vi "READ PORT.vi"(6 "wait for reply (T)":bool=TRUE, 8 "error in (no error)":errorcluster, 10 "CANAL":u8, 11 "Module ID":i32=-1) -> (0 "error out":errorcluster, 1 "timed out?":bool, 2 "Reply Payload":T1)   [LabVIEW 2019, in "MAIN.lvlib"]
doc: "LEE EL PUERTO COMPLETO DE ENTRADAS DE LOS BOTONES, Y LO PASARÁ A UN ARREGLO DE BOOLEANOS\n_____\nCreated using Delacor QMH Event Scripter 5.0.0.112."
uses:
  MAIN.lvlib
  READ PORT (Reply Payload)--cluster.ctl
  READ PORT Argument--cluster.ctl
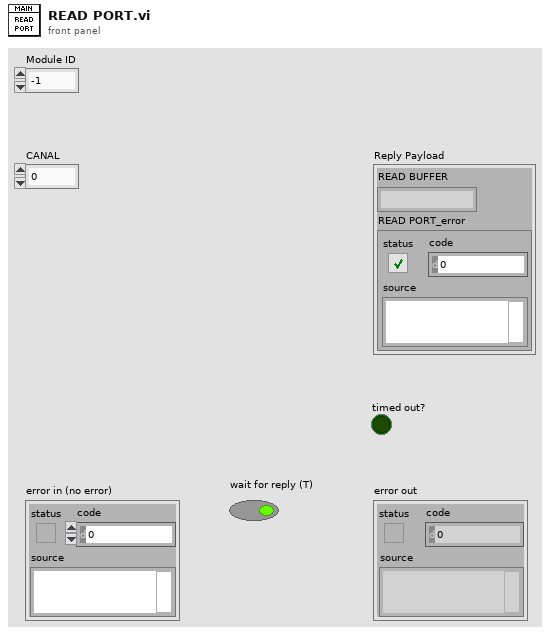
[diagram p1: front panel]
types:
  T1 = typedef "MAIN.lvlib/READ PORT (Reply Payload)--cluster.ctl" = cluster{"READ BUFFER":string, "READ PORT_error":errorcluster}
  T2 = typedef "MAIN.lvlib/READ PORT Argument--cluster.ctl" = cluster{"Module ID":i32, "CANAL":dbl, "Wait Notifier":refnum<notifier>, "wait for reply":bool}
  T3 = typedef "MAIN.lvlib/Request Events--cluster.ctl" = cluster{"Stop Module":refnum<user-event>, "Show Panel":refnum<user-event>, "Hide Panel":refnum<user-event>, "Show Diagram":refnum<user-event>, "Get Module Execution Status":refnum<user-event>, "READ_ADC":refnum<user-event>, "READ PIN":refnum<user-event>, "READ PORT":refnum<user-event>, "WRITE PIN":refnum<user-event>}
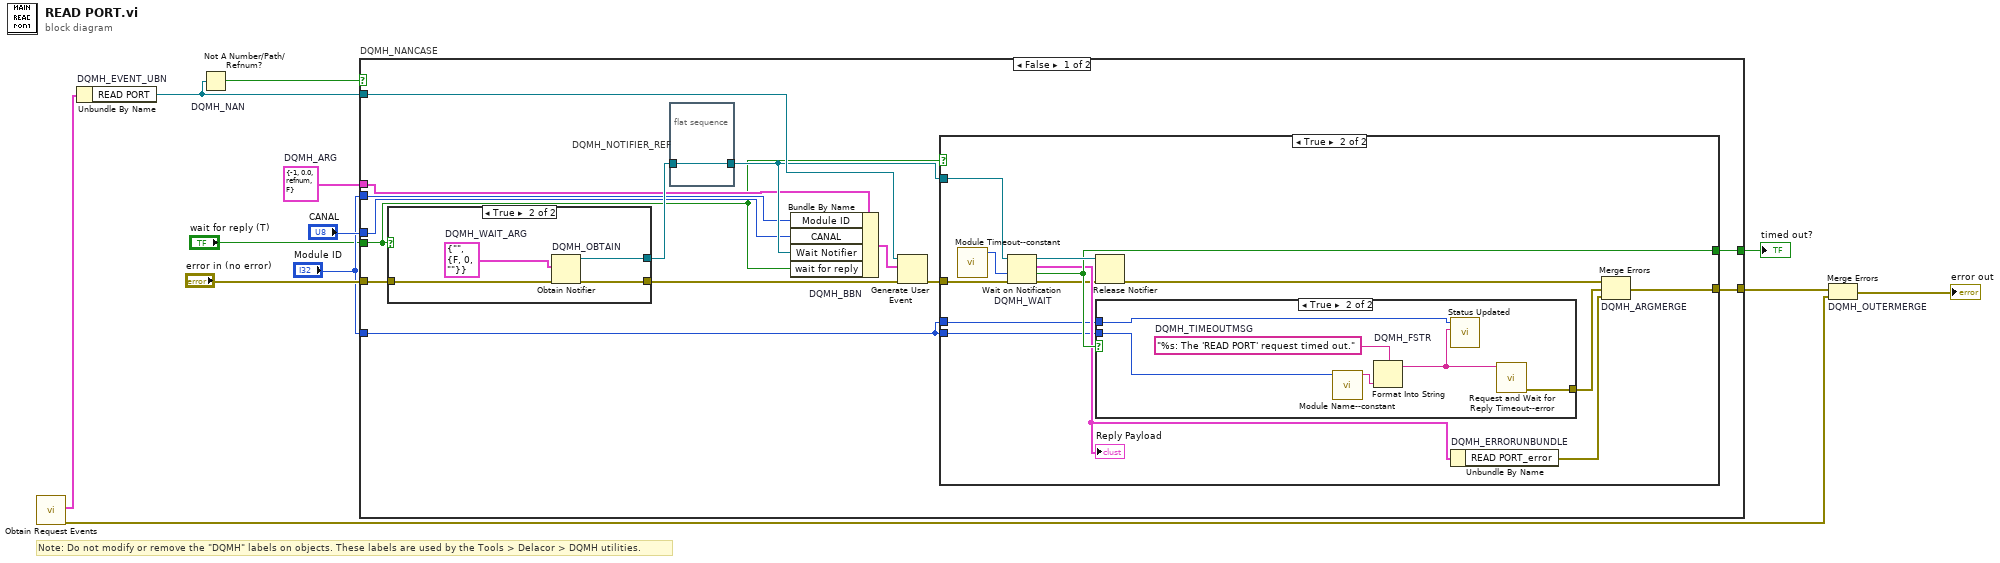
[diagram p0: block diagram]
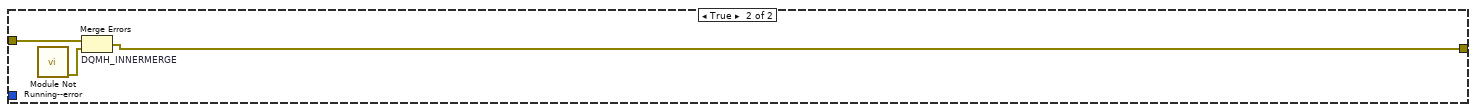
[diagram p5: hidden frame]
diagram:
  w6 = T2 {"Module ID"=-1, "CANAL"=0.0, "Wait Notifier"=refnum, "wait for reply"=FALSE}  # DQMH_ARG
  # "Note: Do not modify or remove the \"DQMH\" labels on objects. These labels are used by the Tools > Delacor > DQMH utilities."
  n1 = call "Obtain Request Events.vi"() -> ("error out"=w2:errorcluster, "MAIN Request Events"=w1:T3)  [unwired: 10 in]
  n2 = Unbundle By Name "DQMH_EVENT_UBN"(w1) -> ("READ PORT"=w10:refnum<user-event>)
  n3 = Not A Number/Path/Refnum? "DQMH_NAN"(number/path/refnum=w10) -> (NaN/Path/Refnum?=w9:bool)
  n4 = case "DQMH_NANCASE" shown="False" w9 {
    tunnel: "error in (no error)" -> [w26 w55]
    tunnel: w10 -> [w24 _]
    tunnel: [w21 w54] -> w7
    tunnel: [w22 _] -> w8
    tunnel: w6 -> [w17 _]
    tunnel: "Module ID" -> [w16 _]
    tunnel: "CANAL" -> [w15 _]
    tunnel: "Module ID" -> [w14 _]
    tunnel: "wait for reply (T)" -> [w13 _]
    frame False {
      n5 = case shown="True" w13 {
        tunnel: w26 -> [w48 w52]
        tunnel: [w48 w51] -> w23
        tunnel: [_ w49] -> w19
        frame False {
        }
        frame True {
          w50 = T1 {"READ BUFFER"="", "READ PORT_error"={"status"=FALSE, "code"=0, "source"=""}}  # DQMH_WAIT_ARG
          n6 = Obtain Notifier "DQMH_OBTAIN"(notification data type=w50, error in (no error)=w52) -> (notifier out=w49:refnum<notifier>, error out=w51:errorcluster)  [unwired: 2 in, 1 out]
        }
      }
      n7 = flat-sequence "DQMH_NOTIFIER_REF" {
        tunnel: w19 -> [w27]
        tunnel: [w27] -> w18
        frame #0 {
        }
      }
      n8 = Bundle By Name "DQMH_BBN"(cluster=w17, "Module ID"=w16, "CANAL"=w15, "Wait Notifier"=w18, "wait for reply"=w13) -> (w20:T2)
      n9 = Generate User Event(user event=w24, event data cluster=w20, error in=w23) -> (error out=w25:errorcluster)  [unwired: 1 in, 1 out]
      n10 = case shown="True" w13 {
        tunnel: w25 -> [w28 w41]
        tunnel: w18 -> [_ w40]
        tunnel: [_ w38] -> w22
        tunnel: [w28 w37] -> w21
        tunnel: w14 -> [_ w30]
        tunnel: w14 -> [_ w29]
        frame False {
        }
        frame True {
          n11 = call "Module Timeout--constant.vi"() -> ("Module Timeout"=w31:i32)  [unwired: 11 in]
          n12 = Wait on Notification "DQMH_WAIT"(notifier=w40, timeout in ms (-1)=w31, error in (no error)=w41) -> (notifier out=w39:refnum<notifier>, notification=w36:T1, timed out?=w38:bool, error out=w35:errorcluster)  [unwired: 1 in]
          "Reply Payload" <- w36
          n13 = Release Notifier(notifier=w39, error in (no error)=w35) -> (error out=w34:errorcluster)  [unwired: 1 in, 2 out]
          n14 = case shown="True" w38 {
            tunnel: [_ w45] -> w32
            tunnel: w30 -> [_ w43]
            tunnel: w29 -> [_ w42]
            frame False {
            }
            frame True {
              w47 = "%s: The 'READ PORT' request timed out."  # DQMH_TIMEOUTMSG
              n15 = call "Module Name--constant.vi"("Module ID"=w42) -> ("Module Name"=w44:string)  [unwired: 10 in]
              n16 = Format Into String "DQMH_FSTR"(format string=w47, w44) -> (resulting string=w46:string)  [unwired: 2 in, 1 out]
              n17 = call "Status Updated.vi"("Status"=w46, "Module ID"=w43) -> ()  [unwired: 9 in, 1 out]
              n18 = call "Request and Wait for Reply Timeout--error.vi"("Error Message"=w46) -> ("error out"=w45:errorcluster)  [unwired: 10 in]
            }
          }
          n19 = Unbundle By Name "DQMH_ERRORUNBUNDLE"(w36) -> ("READ PORT_error"=w33:errorcluster)
          n20 = Merge Errors "DQMH_ARGMERGE"(w34, w32, w33) -> (w37:errorcluster)
        }
      }
    }
    frame True {
      n21 = call "Module Not Running--error.vi"() -> ("error out"=w53:errorcluster)  [unwired: 11 in]
      n22 = Merge Errors "DQMH_INNERMERGE"(w55, w53) -> (w54:errorcluster)
    }
  }
  "timed out?" <- w8
  n23 = Merge Errors "DQMH_OUTERMERGE"(w7, w2) -> (→"error out":errorcluster)
